vi "test_COM.vi"() -> ()   [LabVIEW 2019]
panel:
  out "token":string
  out "error out":errorcluster
  in  "error in":errorcluster {"code" format="%.0x"}
  in  "Порт:":refnum<visa-resource-name>
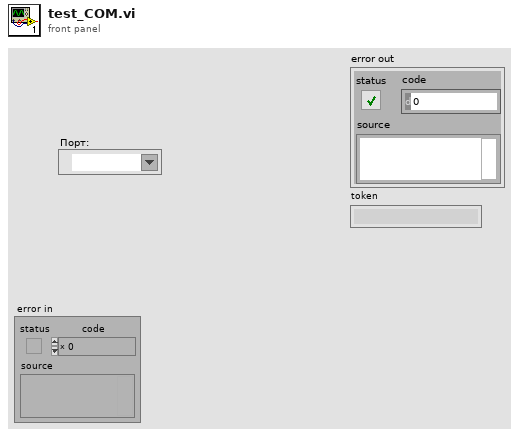
[diagram p1: front panel]
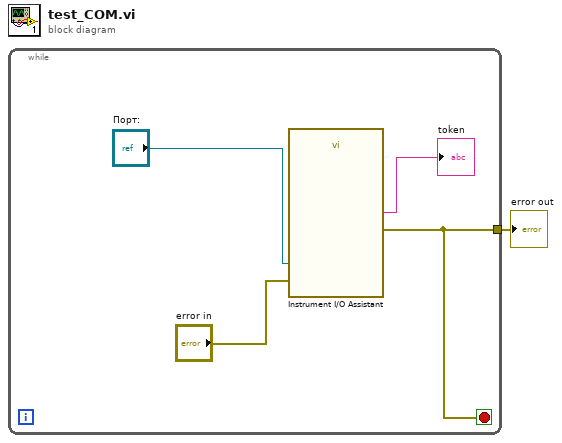
[diagram p0: block diagram]
diagram:
  n1 = while {
    tunnel: [w3] -> w1
    stop <- w3 stop-if-true
    n2 = call "Instrument I/O Assistant"("Session In"="Порт:", "error in"="error in") -> ("token"=→"token":string, "error out"=w3:errorcluster)  [unwired: 23 in, 1 out]
  }
  "error out" <- w1
